vi "myRIOXC Top Level VI Ref.vi"(8 "error in (no error)":errorcluster, 9 "Action":enum16{"Get", "Set"}(ring), 11 "Top Level VI Ref in":refnum<vi>) -> (0 "error out":errorcluster, 3 "Top Level VI Ref out":refnum<vi>)   [LabVIEW 2021]
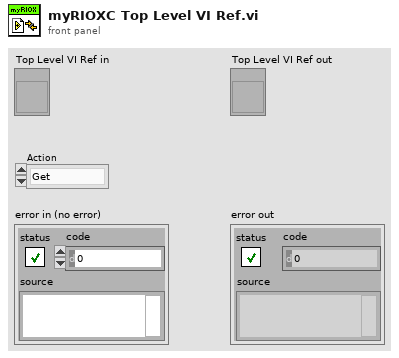
[diagram p1: front panel]
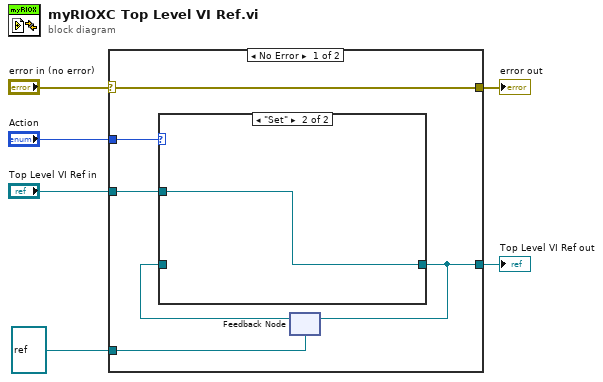
[diagram p0: block diagram]
diagram:
  n1 = case shown="No Error" "error in (no error)" {
    selector: "error in (no error)" -> [w9 w16]
    tunnel: "Action" -> [w12 _]
    tunnel: [w11 w15] -> w1
    tunnel: [w9 w16] -> w4
    tunnel: refnum<vi> refnum ("This VI") -> [w8 w15]
    tunnel: "Top Level VI Ref in" -> [w7 _]
    frame No Error {
      n2 = feedback #1(w8) -> (w10:refnum<vi>)
      n3 = case shown="\"Set\"" w12 {
        tunnel: [w13 w14] -> w11
        tunnel: w10 -> [w13 _]
        tunnel: w7 -> [_ w14]
        frame "Get", Default {
        }
        frame "Set" {
        }
      }
      n4 = feedback-in #1(w11) -> ()
    }
    frame Error {
    }
  }
  "error out" <- w4
  "Top Level VI Ref out" <- w1
